vi "Example MS Chart-Types.vi"() -> ()   [LabVIEW 2015]
uses:
  Controls/Chart.ctl
  Controls/Title.ctl
  Controls/Legend.ctl
  Controls/Series.ctl
  Controls/Marker.ctl
  MSChart/Add Points to Series_DBL[].vi
  Graph Extensions MSChart.lvlib
  System.Windows.Forms.DataVisualization
panel:
  in  "quit":bool
  in  "Scrollbar":i32(c297)=7 caption="Drag this scroll bar to see different plot types."
  in  "ChartType":i32(ring) items=["Point", "FastPoint", "Bubble", "Line", "Spline", "StepLine", "FastLine", "Bar", "StackedBar", "StackedBar100", "Column", "StackedColumn", "StackedColumn100", "Area", "SplineArea", "StackedArea", "StackedArea100", "Pie", "Doughnut", "Stock", "Candlestick", "Range", "SplineRange", "RangeBar", "RangeColumn", "Radar", "Polar", "ErrorBar", "BoxPlot", "Renko", "ThreeLineBreak", "Kagi", "PointAndFigure", "Funnel", "Pyramid"]
  in  "Series":T1={"ChartType"=8, "Name"="chartName", "Palette"=enum."None", "BorderDashStyle"=enum."Solid", "YAxisType"=enum."Secondary", "XAxisType"=enum."Primary", "BorderColor"=0, "Thickness"=1.0, "Color"=16777216, "Alpha"=76, "Marker"={"MarkerStyle"=enum."None", "Size"=12, "Color"=0, "Step"=1}} {"Alpha" scale=0.0..255.0; "ChartType" items=["Point", "FastPoint", "Bubble", "Line", "Spline", "StepLine", "FastLine", "Bar", "StackedBar", "StackedBar100", "Column", "StackedColumn", "StackedColumn100", "Area", "SplineArea", "StackedArea", "StackedArea100", "Pie", "Doughnut", "Stock", "Candlestick", "Range", "SplineRange", "RangeBar", "RangeColumn", "Radar", "Polar", "ErrorBar", "BoxPlot", "Renko", "ThreeLineBreak", "Kagi", "PointAndFigure", "Funnel", "Pyramid"]}
  in  "Data":cluster{"X":dbl, "Y":dbl}[](array[cluster])=[{"X"=0.0, "Y"=0.25}, {"X"=1.0, "Y"=0.75}, {"X"=2.0, "Y"=1.95}, {"X"=3.0, "Y"=1.6}, {"X"=4.0, "Y"=1.6}, {"X"=5.0, "Y"=2.5}, {"X"=6.0, "Y"=1.8}, {"X"=7.0, "Y"=1.26}]
  in  "Chart Options":T3={"ChartName"="Chart4", "BorderDashStyle"=enum."Solid", "Bordercolor"=0, "Title"={"Title"="My TItle", "TitleFontSize"=16.0, "fontName"="Arial", "font Color"=0, "Docking"=enum."Top"}, "Legend"={"Docking"=enum."Top", "BorderDashStyle"=enum."Solid", "BGKcolor"=16646119, "BGKalpha"=134, "Title"="", "TitleSeparator"=enum."None"}} {"Legend"."BGKalpha" scale=0.0..255.0; "Title"."TitleFontSize" min=4.0 max=100.0}
  out "error out":errorcluster
  in  "Chart":refnum<k24>(container)
  # "Instructions:\n1. Setup any chart options and series to the right.  Set any data at the bottom.\n2. Run the VI, then drag the scroll bar to check out all chart types with thaat data and the options.\n3. Stop the VI and rerun, to change data or any chart options and series setup."
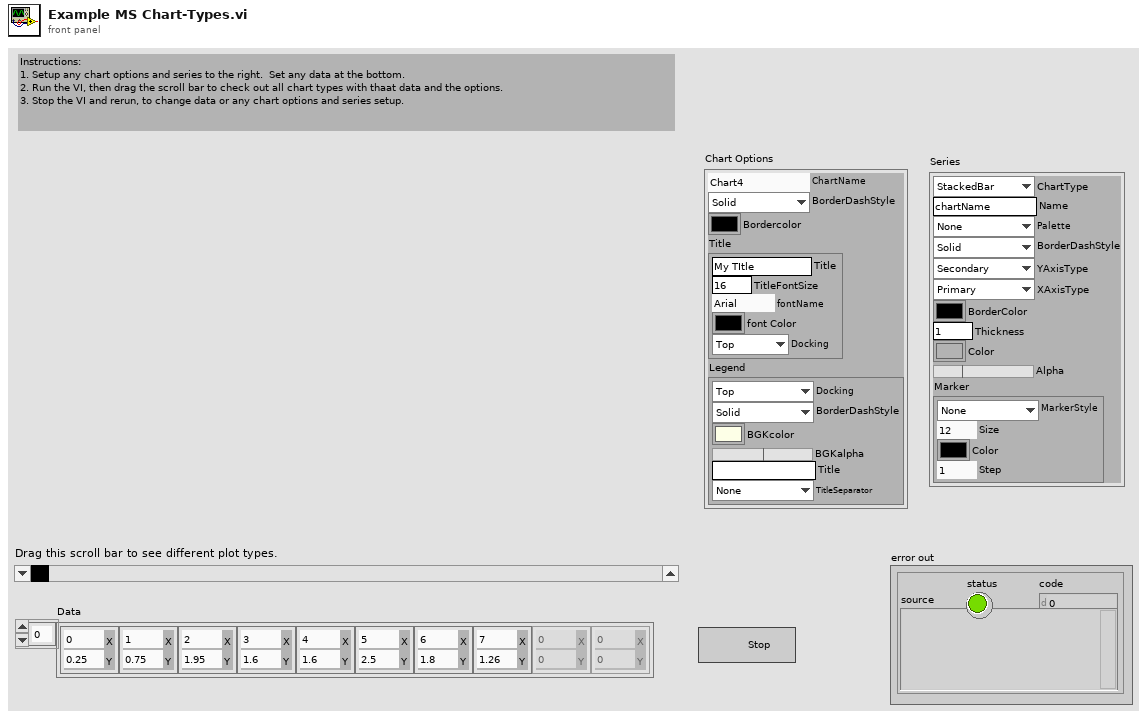
[diagram p1: front panel]
types:
  T1 = typedef "Graph Extensions MSChart.lvlib/Series.ctl" = cluster{"ChartType":i32, "Name":string, "Palette":enum16{"None", "Bright", "Grayscale", "Excel", "Light", "Pastel", "EarthTones", "SemiTransparent", "Berry", "Chocolate", "Fire", "SeaGreen", "BrightPastel"}, "BorderDashStyle":enum16{"NotSet", "Dash", "DashDot", "DashDotDot", "Dot", "Solid"}, "YAxisType":enum16{"Primary", "Secondary"}, "XAxisType":enum16{"Primary", "Secondary"}, "BorderColor":u32, "Thickness":dbl, "Color":u32, "Alpha":u8, "Marker":T2}
  T2 = typedef "Graph Extensions MSChart.lvlib/Marker.ctl" = cluster{"MarkerStyle":enum16{"None", "Square", "Circle", "Diamond", "Triangle", "Cross", "Star4", "Star5", "Star6", "Star10"}, "Size":i32, "Color":u32, "Step":i32}
  T3 = typedef "Graph Extensions MSChart.lvlib/Chart.ctl" = cluster{"ChartName":string, "BorderDashStyle":enum16{"NotSet", "Dash", "DashDot", "DashDotDot", "Dot", "Solid"}, "Bordercolor":u32, "Title":T4, "Legend":T5}
  T4 = typedef "Graph Extensions MSChart.lvlib/Title.ctl" = cluster{"Title":string, "TitleFontSize":dbl, "fontName":string, "font Color":u32, "Docking":enum16{"Top", "Right", "Bottom", "Left"}}
  T5 = typedef "Graph Extensions MSChart.lvlib/Legend.ctl" = cluster{"Docking":enum16{"None", "Top", "Right", "Bottom", "Left"}, "BorderDashStyle":enum16{"NotSet", "Dash", "DashDot", "DashDotDot", "Dot", "Solid"}, "BGKcolor":u32, "BGKalpha":u8, "Title":string, "TitleSeparator":enum16{"None", "Line", "ThickLine", "DoubleLine", "DashLine", "DotLine", "GradientLine", "ThickGradientLine"}}
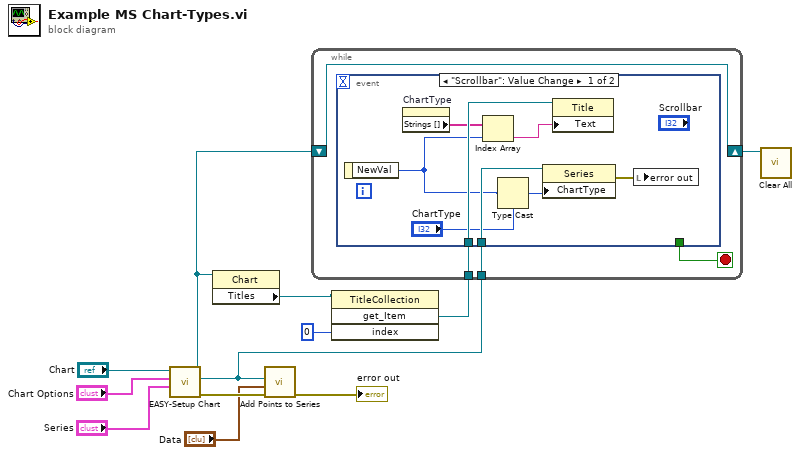
[diagram p0: block diagram]
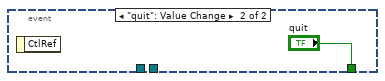
[diagram p2: hidden frame]
diagram:
  n1 = call "EASY-Setup Chart.vi"("Series"="Series", "Chart Options"="Chart Options", ".NET MSChart"="Chart") -> ("error out"=w12:errorcluster, ".net MSChart Series"=w2:refnum<k24>, ".NET MSChart"=w4:refnum<k24>)  [unwired: 6 in]
  n2 = property class="Chart"(reference=w4) -> ("Titles"=w6:refnum<k24>)  [unwired: 1 in, 2 out]
  n3 = call-poly "Add Points to Series.vi"("error in (no error)"=w12, "Data"="Data", ".NET MSChart Series"=w2) -> ("error out"=→"error out":errorcluster)  [unwired: 8 in]
  n4 = invoke class="TitleCollection" method="get_Item"(reference=w6, "index"=0) -> ("get_Item"=w3:refnum<k24>)  [unwired: 2 in, 3 out]
  n5 = while {
    shift-right: [w14] -> w7
    shift-left: w4 -> [w14]
    tunnel: w3 -> [w16]
    tunnel: w2 -> [w15]
    stop <- w13 stop-if-true
    n6 = event shown="[0] \"Scrollbar\": Value Change" {
      selector: _ -> [_ _]
      dyn-events: _ -> [_ _]
      timeout: _ -> [_ _]
      tunnel: w16 -> [w24 _]
      tunnel: w15 -> [w23 _]
      tunnel: [_ "quit"] -> w13
      event "Scrollbar": Value Change {
        n7 = event-data() -> ("NewVal"=w17:i32)  [unwired: 1 in]
        n8 = property on="ChartType" class="Ring (strict)"() -> ("Strings []"=w21:string[])  [unwired: 2 in, 2 out]
        n9 = Index Array(array=w21, index=w17) -> (element=w20:string)
        n10 = Type Cast(type="ChartType", x=w17) -> (*(type *) &x=w18:i32)
        n11 = property class="Series"(reference=w23, "ChartType"=w18) -> (error out=w22:errorcluster)  [unwired: 1 in, 1 out]
        n12 = property class="Title"(reference=w24, "Text"=w20) -> ()  [unwired: 1 in, 2 out]
        n13 = local write "error out"(w22) -> ()
      }
      event "quit": Value Change {
        n14 = event-data() -> ()  [unwired: 1 in, 1 out]
      }
    }
  }
  n15 = call "Clear All.vi"(".NET MSChart ref"=w7) -> ()  [unwired: 11 in]
